vi "Exit While Loop.vi"(0 "Diagram in":refnum<vi>, 1 "Conditional Terminals":refnum<vi>[](array[refnum]), 2 "Loop Terminal Types":T1[](array[typedef]), 5 "Outputs":refnum<vi>[](array[refnum]), 7 "Shift Registers":refnum<vi>[](array[refnum]), 9 "Stop Condition":refnum<vi>, 11 "error in (no error)":errorcluster) -> (4 "Diagram out":refnum<vi>, 6 "Outputs":refnum<vi>[](array[refnum]), 8 "Shift Registers":refnum<vi>[](array[refnum]), 15 "error out":errorcluster)   [LabVIEW 2015, in "Scripting.lvlib"]
doc: "Exits the While Loop that owns <B>Diagram in</B>, supplying the structure's owning diagram at <B>Diagram out</B>.\n\n<B>Stop Condition</B> is the terminal to wire to the conditional terminal of the While Loop.\n\n<B>Conditional Terminals</B> is optionally an array of terminals to wire to the conditional terminal of the While Loop's output tunnels.\n\n<B>Loop Terminal Types</B> is optionally and array of terminal types of the While Loop's output tunnels."
uses:
  Scripting.lvlib
  Loop Terminal Type.ctl
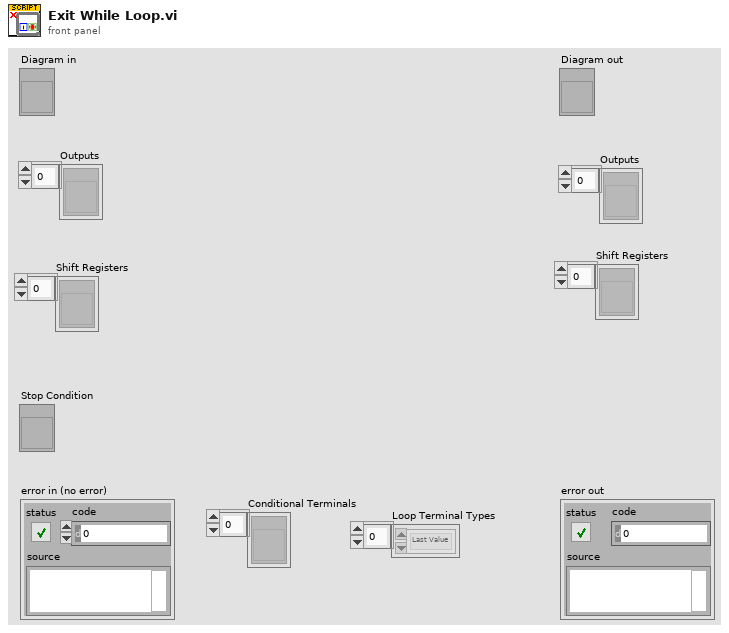
[diagram p1: front panel]
types:
  T1 = typedef "Scripting.lvlib/Loop Terminal Type.ctl" = enum16{"Last Value", "Indexing", "Concatenating"}
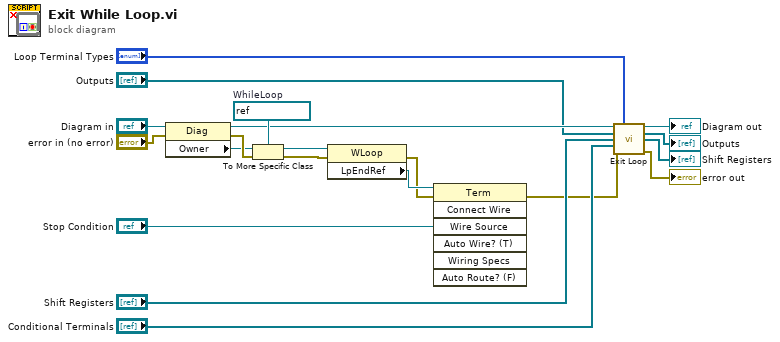
[diagram p0: block diagram]
diagram:
  w19 = refnum<vi> refnum  # WhileLoop
  n1 = property class="Diag"(reference="Diagram in", error in="error in (no error)") -> (reference out=w15:refnum<vi>, error out=w20:errorcluster, "Owner"=w18:refnum<vi>)
  n2 = To More Specific Class(target class=w19, reference=w18, error in=w20) -> (specific class reference=w9:refnum<vi>, error out=w8:errorcluster)
  n3 = property class="WLoop"(reference=w9, error in=w8) -> (error out=w2:errorcluster, "LpEndRef"=w3:refnum<vi>)  [unwired: 1 out]
  n4 = invoke class="Term" method="Connect Wire"(reference=w3, error in=w2, "Wire Source"="Stop Condition") -> (error out=w5:errorcluster)  [unwired: 4 in, 6 out]
  n5 = call "Exit Loop.vi"("Diagram in"=w15, "Loop Terminal Types"="Loop Terminal Types", "Outputs"="Outputs", "Shift Registers"="Shift Registers", "Conditional Terminals"="Conditional Terminals", "error in (no error)"=w5) -> ("Diagram out"=→"Diagram out":refnum<vi>, "Outputs"=→"Outputs":refnum<vi>[], "Shift Registers"=→"Shift Registers":refnum<vi>[], "error out"=→"error out":errorcluster)  [unwired: 6 in]
